vi "Write File Refnum.vi"(8 "error in (no error)":errorcluster, 10 "file refnum":refnum<file>, 11 "read file in":refnum<class "Read File.lvclass">) -> (0 "error out":errorcluster, 3 "read file out":refnum<class "Read File.lvclass">)   [LabVIEW 2023, in "read file.lvclass"]
doc: "Sets a file reference number to Read File.ctl."
uses:
  Read File.lvclass
  Read File.lvclass/Read File.ctl
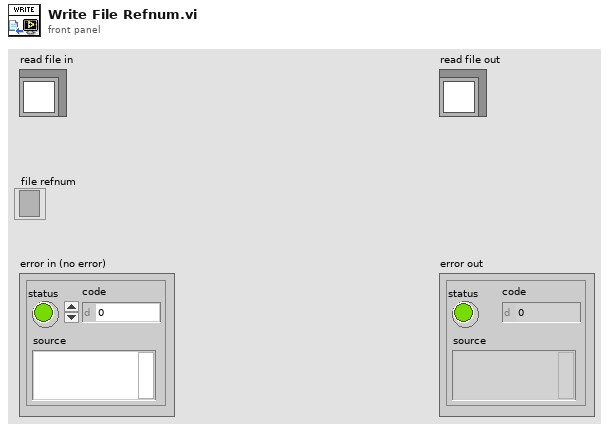
[diagram p1: front panel]
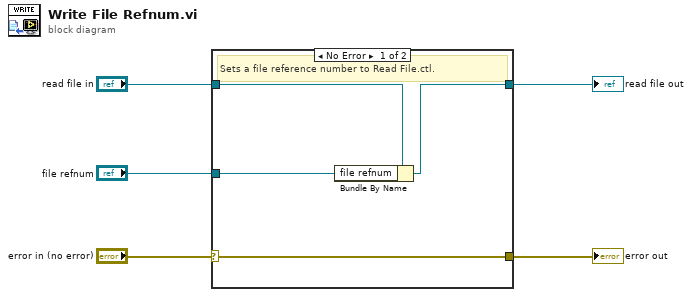
[diagram p0: block diagram]
diagram:
  n1 = case shown="No Error" "error in (no error)" {
    selector: "error in (no error)" -> [w9 w10]
    tunnel: [w9 w10] -> w4
    tunnel: [w7 w11] -> w2
    tunnel: "read file in" -> [w8 w11]
    tunnel: "file refnum" -> [w6 _]
    frame No Error {
      # "Sets a file reference number to Read File.ctl."
      n2 = Bundle By Name(cluster=w8, "file refnum"=w6) -> (w7:refnum<class "Read File.lvclass">)
    }
    frame Error {
    }
  }
  "error out" <- w4
  "read file out" <- w2
